vi "GIF.Write.Pack.Data__ogtk.vi"(6 "Delay (ms)":u32, 8 "error in (no error)":errorcluster, 11 "LV image data":T1) -> (0 "error out":errorcluster, 3 "Pack in-progress out":u8[](array[numeric]))   [LabVIEW 2011]
uses:
  <vilib>/picture/picture.llb/imagedata.ctl
panel:
  # "GIF.Write.Pack.Datavi\n\nBuilds GIF Data section.  A GIF can contain multiple Data sections.\n\nPlease visit http://www.OpenG.org to learn about the\nOpen Source LabVIEW software movement.\n\nNOTICE -- YOU MUST LEAVE THIS NOTICE IN PLACE.  PER THE TERMS OF THE LICENSE BELOW, YOU MAY SUBLICENSE THIS SOFTWARE \nIN ANY WAY THAT DOES NOT CONFLICT WITH THIS LICENSE.\n\n### BSD License (http://www.opensource.org/licenses/bsd-license.php) Begin ###\n \nCopyright (c) 2007, Bill Clench <bclench@yahoo.com>\n\nAll rights reserved.\n\nRedistribution and use in source and binary forms, with or without modification, are permitted provided that the following conditions are met:\n\n    * Redistributions of source code must retain the above copyright notice, this list of conditions and the following disclaimer.\n    * Redistributions in binary form must reproduce the above copyright notice, this list of conditions and the following disclaimer in the \n       documentation and/or other materials provided with the distribution.\n    * Neither the name of SciWare, James Kring, Inc., nor the names of its contributors may be used to endorse or promote products derived \n       from this software without specific prior written permission.\n\nTHIS SOFTWARE IS PROVIDED BY THE COPYRIGHT HOLDERS AND CONTRIBUTORS \"AS IS\" AND ANY EXPRESS OR IMPLIED WARRANTIES, \nINCLUDING, BUT NOT LIMITED TO, THE IMPLIED WARRANTIES OF MERCHANTABILITY AND FITNESS FOR A PARTICULAR PURPOSE ARE \nDISCLAIMED. IN NO EVENT SHALL THE COPYRIGHT OWNER OR CONTRIBUTORS BE LIABLE FOR ANY DIRECT, INDIRECT, INCIDENTAL,\n SPECIAL, EXEMPLARY, OR CONSEQUENTIAL DAMAGES (INCLUDING, BUT NOT LIMITED TO, PROCUREMENT OF SUBSTITUTE GOODS OR \nSERVICES; LOSS OF USE, DATA, OR PROFITS; OR BUSINESS INTERRUPTION) HOWEVER CAUSED AND ON ANY THEORY OF LIABILITY, \nWHETHER IN CONTRACT, STRICT LIABILITY, OR TORT (INCLUDING NEGLIGENCE OR OTHERWISE) ARISING IN ANY WAY OUT OF THE USE \nOF THIS SOFTWARE, EVEN IF ADVISED OF THE POSSIBILITY OF SUCH DAMAGE.\n\n### BSD License End ###"
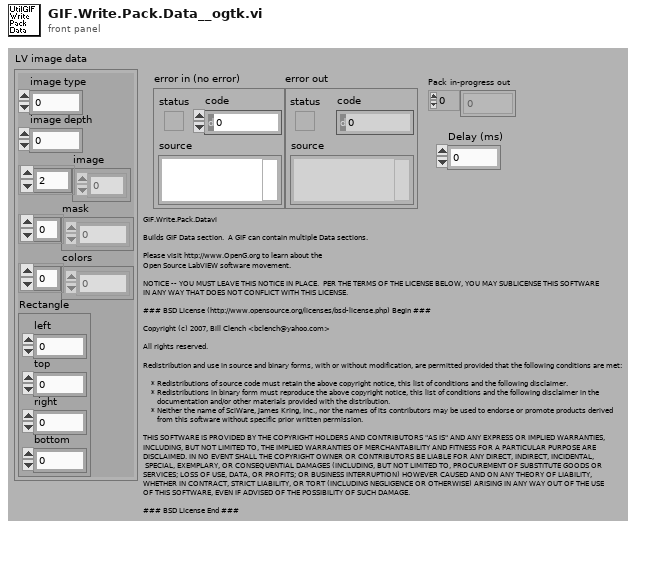
[diagram p1: front panel]
types:
  T1 = typedef "imagedata.ctl" = cluster{"image type":i32, "image depth":i32, "image":u8[], "mask":u8[], "colors":u32[], "Rectangle":cluster{"left":i16, "top":i16, "right":i16, "bottom":i16}}
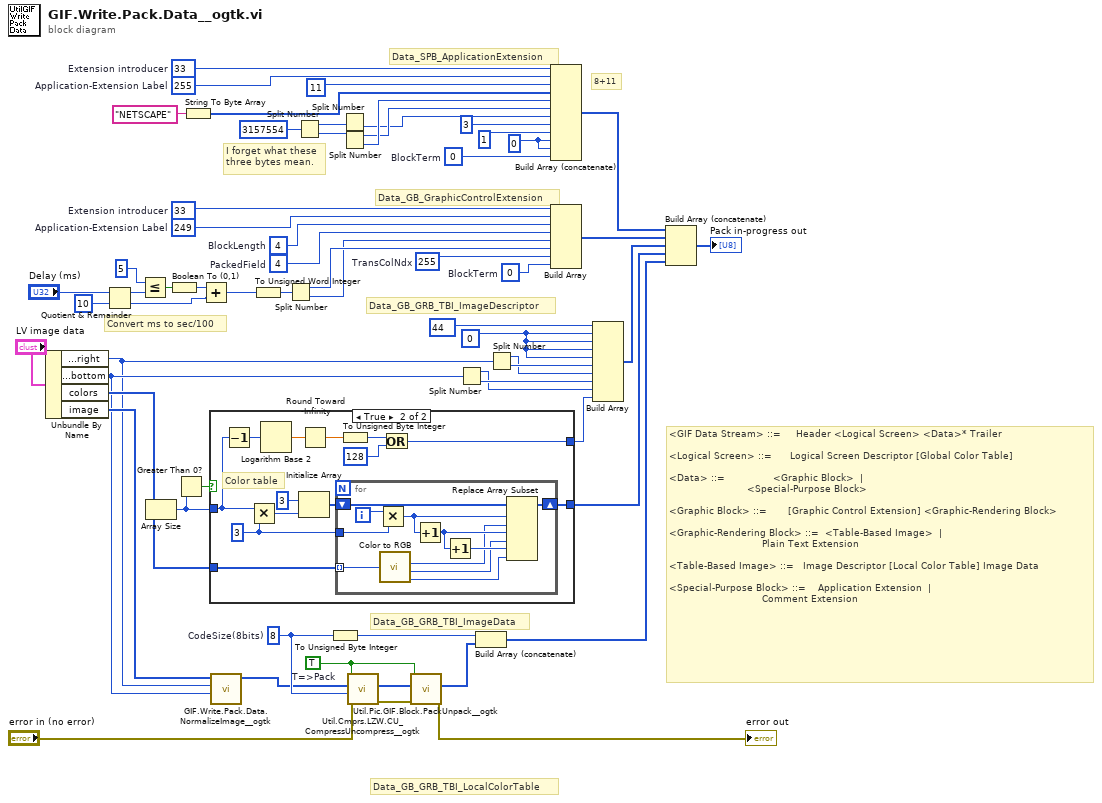
[diagram p0: block diagram]
diagram:
  w22 = TRUE  # T=>Pack
  w16 = 8  # CodeSize(8bits)
  w31 = u8 0
  w43 = u8 0  # BlockTerm
  w42 = u8 255  # TransColNdx
  w38 = u8 4  # PackedField
  w37 = u8 4  # BlockLength
  w36 = u8 249  # Application-Extension Label
  w35 = u8 33  # Extension introducer
  w49 = u8 0 ("element")
  w48 = u8 0  # BlockTerm
  w47 = u8 255  # Application-Extension Label
  w61 = u8 33  # Extension introducer
  # "Convert ms to sec/100"
  # "8+11"
  # "Data_GB_GRB_TBI_ImageData"
  # "I forget what these\nthree bytes mean."
  # "Data_GB_GRB_TBI_LocalColorTable"
  # "Data_GB_GRB_TBI_ImageDescriptor"
  # "Data_GB_GraphicControlExtension"
  # "<GIF Data Stream> ::=     Header <Logical Screen> <Data>* Trailer\n\n<Logical Screen> ::=      Logical Screen Descriptor [Global Color Table]\n\n<Data> ::=                <Graphic Block>  |\n                          <Special-Purpose Block>\n\n<Graphic Block> ::=       [Graphic Control Extension] <Graphic-Rendering Block>\n\n<Graphic-Rendering Block> ::=  <Table-Based Image>  |\n                               Plain Text Extension\n\n<Table-Based Image> ::=   Image Descriptor [Local Color Table] Image Data\n\n<Special-Purpose Block> ::=    Application Extension  |\n                               Comment Extension"
  # "Data_SPB_ApplicationExtension"
  n1 = Unbundle By Name("LV image data") -> ("Rectangle.right"=w1:i16, "Rectangle.bottom"=w2:i16, "colors"=w46:u32[], "image"=w3:u8[])
  n2 = Quotient & Remainder(x="Delay (ms)", y=u32 10) -> (x-y*floor(x/y)=w10:u32, floor(x/y)=w6:u32)
  n3 = Less Or Equal?(x=u8 5, y=w10) -> (x <= y?=w8:bool)
  n4 = Array Size(array=w46) -> (size(s)=w45:i32)
  n5 = Boolean To (0,1)(Boolean=w8) -> (0, 1=w7:i16)
  n6 = Greater Than 0?(x=w45) -> (x > 0?=w15:bool)
  n7 = String To Byte Array(string="NETSCAPE") -> (unsigned byte array=w58:u8[])
  n8 = Add(x=w7, y=w6) -> (x+y=w5:u32)
  n9 = case shown="True" w15 {
    tunnel: [_ w70] -> w25
    tunnel: w46 -> [_ w69]
    tunnel: w45 -> [_ w68]
    tunnel: [_ w63] -> w14
    frame False {
    }
    frame True {
      w74 = 3 ("y")
      # "Color table"
      n10 = Decrement(x=w68) -> (x-1=w67:i32)
      n11 = Multiply(x=w68, y=w74) -> (x*y=w72:i32)
      n12 = Logarithm Base 2(1:w67) -> (0:w66:dbl)
      n13 = Initialize Array(u8 3 ("y"), w72) -> (w71:u8[])
      n14 = Round Toward -Infinity(1:w66) -> (0:w62:dbl)
      n15 = for {
        shift-right: [w84] -> w70
        shift-left: w71 -> [w85]
        tunnel: w69 -> [w78] mode=indexing
        tunnel: w74 -> [w82]
        i -> [w83]
        n16 = Multiply(x=w83, y=w82) -> (x*y=w81:i32)
        n17 = call <vilib>:"Color to RGB.vi"("Color"=w78) -> ("R"=w77:u8, "G"=w76:u8, "B"=w75:u8)  [unwired: 1 out]
        n18 = Increment(x=w81) -> (x+1=w80:i32)
        n19 = Increment(x=w80) -> (x+1=w79:i32)
        n20 = Replace Array Subset(array=w85, new element #1=w77, index #1=w81, new element #2=w76, index #2=w80, new element #3=w75, index #3=w79) -> (w84:u8[])
      }
      n21 = To Unsigned Byte Integer(number=w62) -> (unsigned 8bit integer=w65:u8)
      n22 = Or(x=w65, y=u8 128) -> (x .or. y?=w63:u8)
    }
  }
  n23 = call "GIF.Write.Pack.Data.NormalizeImage__ogtk.vi"("bottom"=w2, "right"=w1, "ImageIn"=w3) -> ("ImageOut"=w4:u8[])  [unwired: 8 in]
  n24 = To Unsigned Word Integer(number=w5) -> (unsigned 16bit integer=w39:u16)
  n25 = Split Number(x=w39) -> (hi(x)=w41:u8, lo(x)=w40:u8)
  n26 = Split Number(x=u32 3157554) -> (hi(x)=w56:u16, lo(x)=w55:u16)
  n27 = To Unsigned Byte Integer(number=w16) -> (unsigned 8bit integer=w12:u8)
  n28 = Split Number(x=w56) -> (lo(x)=w52:u8)  [unwired: 1 out]
  n29 = Split Number(x=w55) -> (hi(x)=w53:u8, lo(x)=w54:u8)
  n30 = call "Util.Cmprs.LZW.CU_CompressUncompress__ogtk.vi"("error in (no error)"="error in (no error)", "LZWBits"=w16, "Data"=w4, "Compress/Decompress (T/F)"=w22) -> ("error out"=w20:errorcluster, "Data out"=w17:u8[])  [unwired: 6 in]
  n31 = call "Util.Pic.GIF.Block.PackUnpack__ogtk.vi"("error in (no error)"=w20, "BlockBytes in"=w17, "Pack/Unpack (T/F)"=w22) -> ("error out"=→"error out":errorcluster, "BlockBytes out"=w18:u8[])  [unwired: 6 in, 1 out]
  n32 = Split Number(x=w2) -> (hi(x)=w27:u8, lo(x)=w28:u8)
  n33 = Build Array (concatenate)(w12, w18) -> (w23:u8[])
  n34 = Split Number(x=w1) -> (hi(x)=w29:u8, lo(x)=w30:u8)
  n35 = Build Array (concatenate)(w61, w47, u8 11, w58, w54, w53, w52, u8 3 ("element"), u8 1 ("element"), w49, w49, w48) -> (w44:u8[])
  n36 = Build Array(w35, w36, w37, w38, w40, w41, w42, w43) -> (w33:u8[])
  n37 = Build Array(u8 44, w31, w31, w31, w31, w30, w29, w28, w27, w14) -> (w26:u8[])
  n38 = Build Array (concatenate)(w44, w33, w26, w25, w23) -> (→"Pack in-progress out":u8[])
